vi "HapticSTM_Feedblackless.vi"() -> ()   [LabVIEW 2019]
uses:
  <userlib>/HapticSTM/GlobalClicksHeight.vi
  <userlib>/HapticSTM/HapticSTM.lvlib
  <instrlib>/Nanonis Prog Interface V5/Nanonis Prog Interface.lvlib
panel:
  out "Button":bool
  out "Zpos":cluster{dbl, "Y":dbl, i16}(graph)
  out "Filtered Current (pA)":dbl
  in  "Reset Clicks":bool
  out "Scaled Force and Current":cluster{dbl, "Filtered x":dbl, dbl}(graph)
  in  "Maximum (pA)":dbl=5000.0
  out "Plane Height (m)":dbl
  out "Raw Current (pA)":dbl
  out "Origin Y (nm)":dbl
  out "Origin X (nm)":dbl
  out "Output Z":dbl
  in  "Rough adjust":dbl
  out "Nano Z Write (m)":dbl
  out "Width (nm)":dbl
  out "VY":dbl
  out "VZ":dbl
  out "VX":dbl
  in  "Drag":dbl=1.0
  in  "STOP":bool
  in  "START":bool
  out "Fy (N)":dbl
  out "Fz (N)":dbl
  out "phi":dbl
  out "psi":dbl
  out "Fx (N)":dbl
  out "theta":dbl
  out "x (nm)":dbl
  out "y (mm)":dbl
  out "z (nm)":dbl
  in  "Fine adjust":dbl=3.5
  out "Clicks":dbl
  out "Height (nm)":dbl
  # "Sample Window"
  # "Position"
  # "Sensitivity"
  # "Force"
  # "STM I/O"
  # "Angles"
  # "Current"
  # "Velocity"
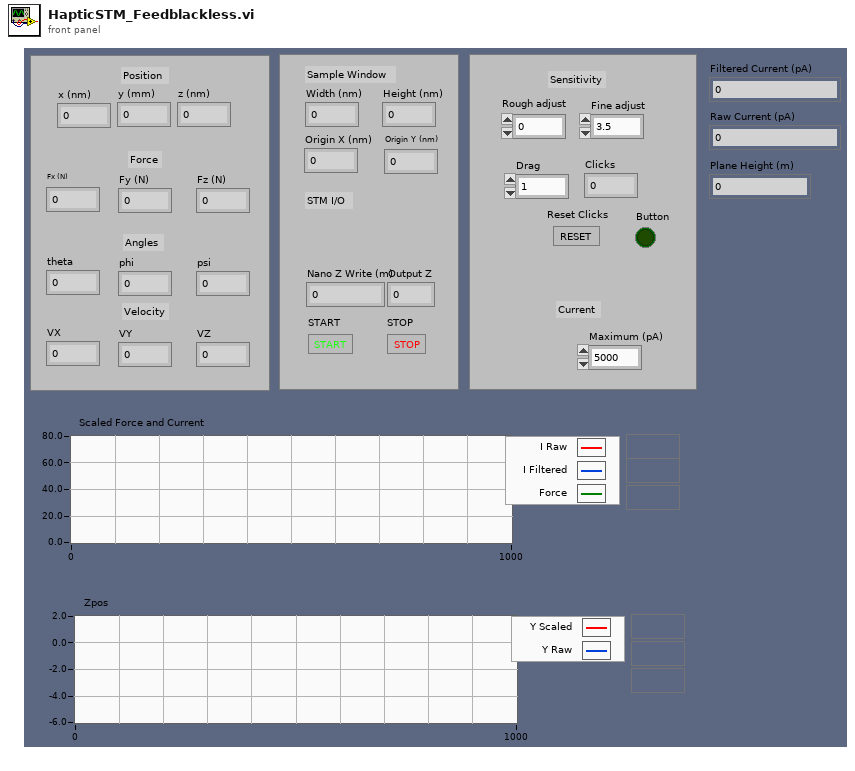
[diagram p1: front panel]
types:
  T1 = cluster{"Center coordinates (m)":cluster{"Xc":sgl, "Yc":sgl}, "Size (m)":cluster{"Width":sgl, "Height":sgl}}
  T2 = cluster{"Raw Current (pA)":dbl, "Filtered Current (pA)":dbl, dbl}
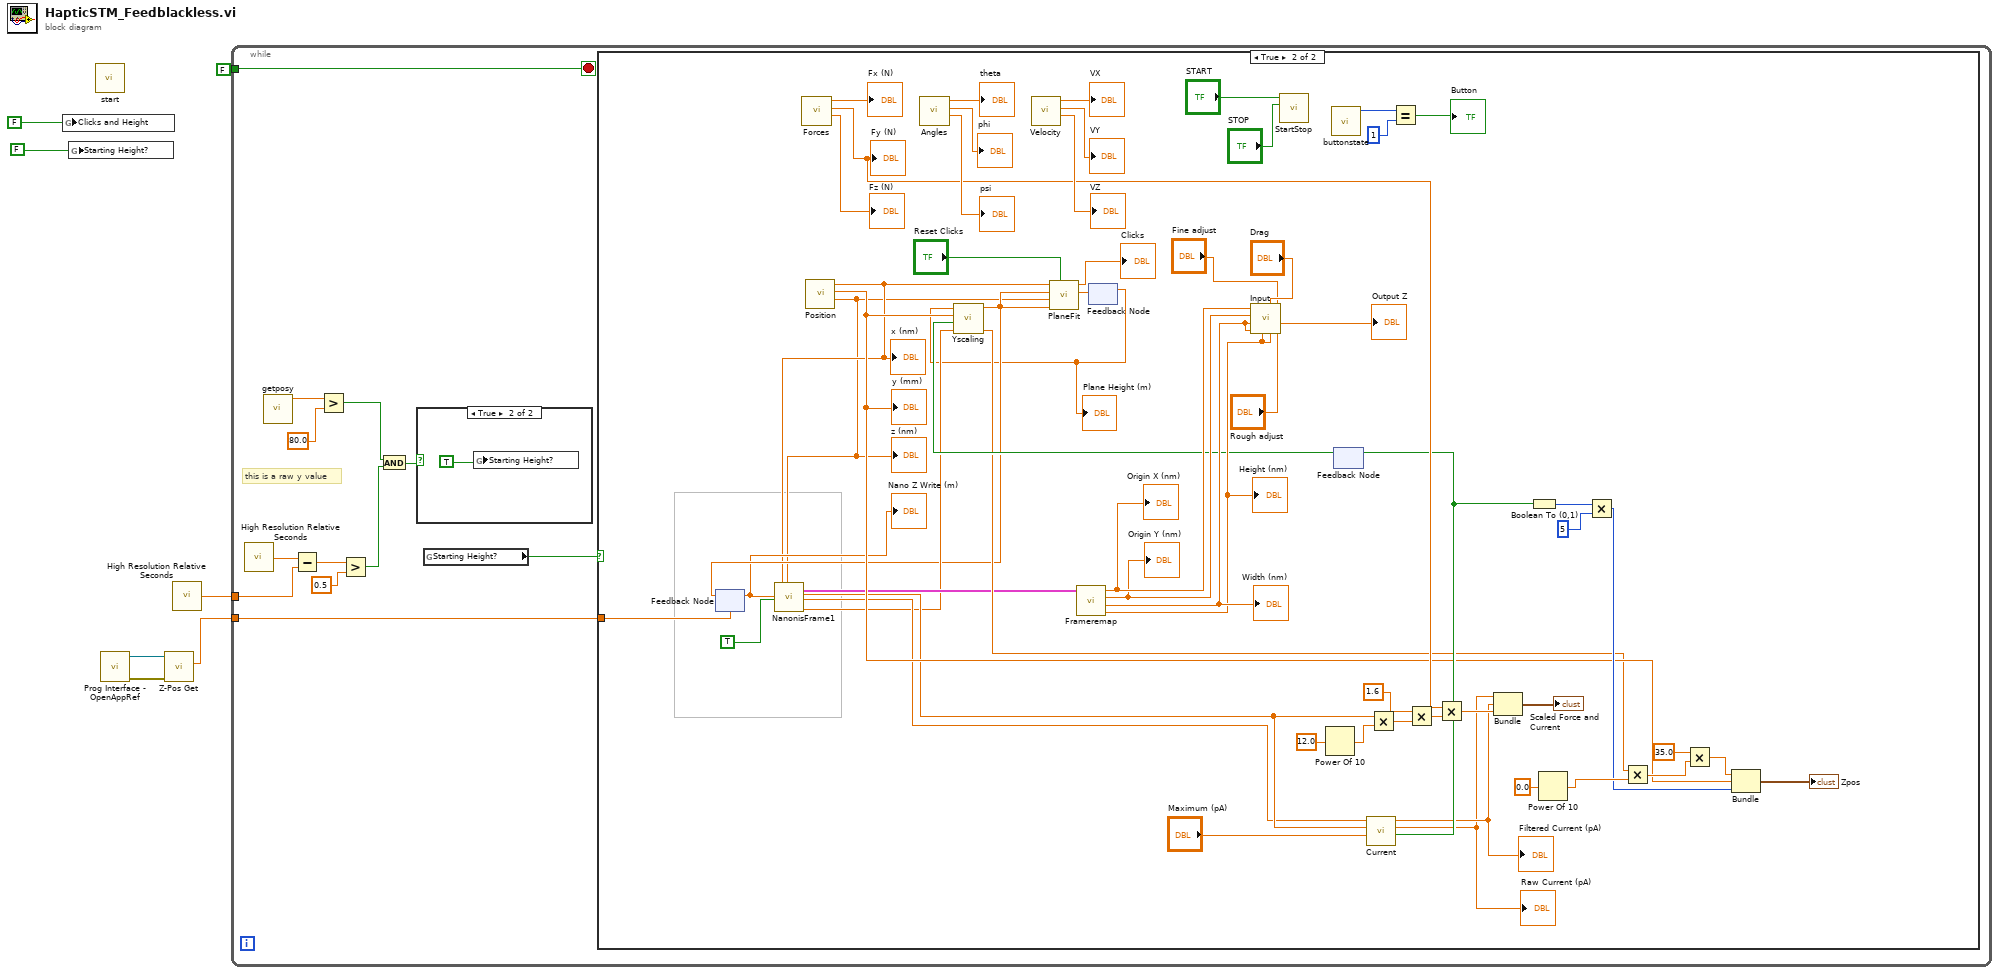
[diagram p0: block diagram]
diagram:
  n1 = global write "GlobalClicksHeight.vi" "Clicks and Height"(FALSE ("Clicks and Height")) -> ()
  n2 = global write "GlobalClicksHeight.vi" "Starting Height?"(FALSE ("Clicks and Height")) -> ()
  n3 = call <userlib>:"start.vi"() -> ()  [unwired: 11 in, 1 out]
  n4 = call <instrlib>:"Prog Interface - OpenAppRef.vi"() -> ("Error out"=w3:errorcluster, "Application reference"=w2:refnum<vi>)  [unwired: 6 in]
  n5 = call <instrlib>:"Z-Pos Get.vi"("error in (no error)"=w3, "Application ref in"=w2) -> ("Z position (m)"=w1:sgl)  [unwired: 7 in, 2 out]
  n6 = call <vilib>:"High Resolution Relative Seconds.vi"() -> ("relative seconds"=w4:dbl)
  n7 = while {
    tunnel: FALSE -> [w19]
    tunnel: w4 -> [w12]
    tunnel: w1 -> [w11]
    stop <- w19 stop-if-true
    # "this is a raw y value"
    n8 = call <vilib>:"High Resolution Relative Seconds.vi"() -> ("relative seconds"=w13:dbl)
    n9 = call <userlib>:"getposy.vi"() -> ("function return"=w18:dbl)  [unwired: 11 in]
    n10 = Subtract(x=w13, y=w12) -> (x-y=w10:dbl)
    n11 = Greater?(x=w18, y=80.0) -> (0:w14:bool)
    n12 = Greater?(x=w10, y=0.5) -> (0:w8:bool)
    n13 = And(x=w14, y=w8) -> (x .and. y?=w15:bool)
    n14 = case shown="True" w15 {
      frame False {
      }
      frame True {
        n15 = global write "GlobalClicksHeight.vi" "Starting Height?"(TRUE ("Clicks and Height")) -> ()
      }
    }
    n16 = global read "GlobalClicksHeight.vi" "Starting Height?"() -> (w16:bool)
    n17 = case shown="True" w16 {
      tunnel: w11 -> [_ w27]
      frame False {
      }
      frame True {
        n18 = feedback #1(w27) -> (w25:dbl)
        "Nano Z Write (m)" <- w25
        n19 = call <userlib>:"Forces.vi"() -> ("Fz"=→"Fz (N)":dbl, "Fy"=w56:dbl, "Fx"=→"Fx (N)":dbl)  [unwired: 9 in]
        "Fy (N)" <- w56
        n20 = call <userlib>:"Position.vi"() -> ("Z"=w23:dbl, "Y"=w36:dbl, "X"=w24:dbl)  [unwired: 9 in]
        "x (nm)" <- w24
        "y (mm)" <- w36
        "z (nm)" <- w23
        n21 = call <userlib>:"NanonisFrame1.vi"("Nano Z Write (m)"=w25, "Begin Writing?"=TRUE, "x (nm)"=w24, "z (nm)"=w23) -> ("Frame Parameters (m)"=w31:T1, "Setpoint Current (A)"=w30:dbl, "Current (A)"=w29:dbl, "Nano Z Read (m)"=w28:sgl)  [unwired: 11 in, 1 out]
        n22 = call <userlib>:"Angles.vi"() -> ("psi"=→"psi":dbl, "phi"=→"phi":dbl, "theta"=→"theta":dbl)  [unwired: 9 in]
        n23 = call <userlib>:"Velocity.vi"() -> ("VZ"=→"VZ":dbl, "VY"=→"VY":dbl, "VX"=→"VX":dbl)  [unwired: 9 in]
        n24 = call <userlib>:"Frameremap.vi"("Frame Parameters (m)"=w31) -> ("FH (nm)"=w66:dbl, "FW (nm)"=w67:dbl, "Z Origin (nm)"=w60:dbl, "X Origin (nm)"=w61:dbl)  [unwired: 7 in]
        "Height (nm)" <- w66
        "Width (nm)" <- w67
        "Origin X (nm)" <- w61
        "Origin Y (nm)" <- w60
        n25 = feedback #2() -> (w21:dbl)  [unwired: 1 in]
        "Plane Height (m)" <- w21
        n26 = call <userlib>:"Input.vi"("Current * 10^input"="Rough adjust", "Sensitivity"="Fine adjust", "Scopez"=w66, "Drag"="Drag", "FH"=w66, "FW"=w67, "Scopex"=w67, "Z origin"=w60, "X origin"=w61) -> ("Scaled Current"=→"Output Z":dbl)  [unwired: 2 in]
        n27 = call <userlib>:"StartStop.vi"("STOP"="STOP", "START"="START") -> ()  [unwired: 10 in]
        n28 = Power Of 10(x=12.0) -> (10^x=w59:dbl)
        n29 = call <userlib>:"buttonstate.vi"() -> ("function return"=w46:i32)  [unwired: 11 in]
        n30 = feedback #3() -> (w35:bool)  [unwired: 1 in]
        n31 = call <userlib>:"Yscaling.vi"("Nano Z Read (m)"=w28, "Current Maxed?"=w35, "Y"=w36, "Plane Height"=w21) -> ("y scaled (nm)"=w34:dbl, "Nano Z Write (m)"=w26:dbl)  [unwired: 5 in]
        n32 = feedback-in #1(w26) -> ()
        n33 = call <userlib>:"PlaneFit.vi"("Reset Clicks"="Reset Clicks", "Y PEN"=w26, "Z"=w23, "Nano Z"=w26, "X"=w24) -> ("Plane Height (m)"=w62:dbl, "Clicks"=→"Clicks":dbl)  [unwired: 5 in]
        n34 = feedback-in #2(w62) -> ()
        n35 = call <userlib>:"Current.vi"("Maximum Current (pA)"="Maximum (pA)", "Setpoint Current (A)"=w30, "Current (A)"=w29) -> ("Current Maxed?"=w39:bool, "Raw Current (pA)"=w32:dbl, "Filtered Current (pA)"=w33:dbl)  [unwired: 6 in]
        "Raw Current (pA)" <- w32
        "Filtered Current (pA)" <- w33
        n36 = feedback-in #3(w39) -> ()
        n37 = Multiply(x=w30, y=w59) -> (x*y=w37:dbl)
        n38 = Equal?(x=w46, y=1) -> (x = y?=→"Button":bool)
        n39 = Multiply(x=1.6 ("y"), y=w37) -> (x*y=w40:dbl)
        n40 = Multiply(x=w56, y=w40) -> (x*y=w55:dbl)
        n41 = Bundle("Raw Current (pA)"=w32, "Filtered Current (pA)"=w33, w55) -> (→"Scaled Force and Current":T2)  [unwired: 1 in]
        n42 = Boolean To (0,1)(Boolean=w39) -> (0, 1=w43:i16)
        n43 = Power Of 10(x=0.0) -> (10^x=w52:dbl)
        n44 = Multiply(x=w43, y=i16 5) -> (x*y=w41:i16)
        n45 = Multiply(x=w34, y=w52) -> (x*y=w48:dbl)
        n46 = Multiply(x=35.0, y=w48) -> (x*y=w49:dbl)
        n47 = Bundle(w49, "Y"=w36, w41) -> (→"Zpos":cluster{dbl, "Y":dbl, i16})  [unwired: 1 in]
      }
    }
  }
